vi "copy directory contents.vi"(2 "error in":errorcluster, 3 "target directory":path=path "\\\\Enviro\\enviro/Software/RunTime7", 4 "Source directory":path=path "\\\\Enviro\\enviro/Software/RunTime7") -> (0 "error out":errorcluster)   [LabVIEW 2010]
panel:
  out "Current file":string
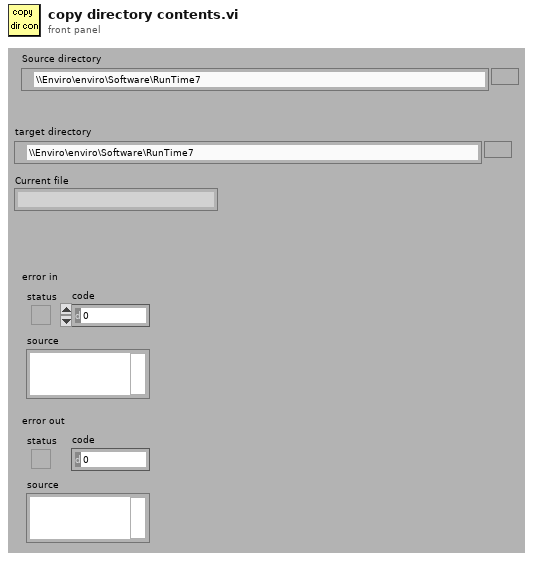
[diagram p1: front panel]
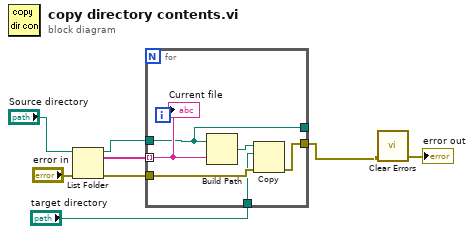
[diagram p0: block diagram]
diagram:
  n1 = List Folder(path="Source directory", error in="error in") -> (path out=w4:path, filenames=w8:string[], error out=w7:errorcluster)  [unwired: 2 in, 1 out]
  n2 = for {
    tunnel: w4 -> [w12]
    tunnel: w8 -> [w13] mode=indexing
    tunnel: [w12] -> _
    tunnel: [w11] -> w3
    tunnel: w7 -> [w10]
    tunnel: "target directory" -> [w9]
    n3 = Build Path(base path=w12, name or relative path=w13) -> (appended path=w14:path)
    n4 = Copy(8:w10, 10:w9, 11:w14) -> (0:w11:errorcluster)  [unwired: 2 in, 2 out]
    "Current file" <- w13
  }
  n5 = call <vilib>:"Clear Errors.vi"("error in (no error)"=w3) -> ("error out"=→"error out":errorcluster)  [unwired: 6 in]
